vi "参数设置页.vi"() -> ()   [LabVIEW 2016, in "斯坦道氨氮.lvlib"]
uses:
  <vilib>/Plasmionique/MB Master/MB_Master/MB_Master.lvclass
  <vilib>/ptbypt/NI_PtbyPt.lvlib
panel:
  in  "简易流程路径":path=path "data/流程.xml"
  out "数据刷新时间":string
  in  "通讯连接":bool
  out "MB table":enum32{"Serial", "TCP"}(tab)
  in  "请选择串口:":refnum<visa-resource-name>
  in  "IP":string="127.0.0.1"
  in  "PORT":string="1001"
  in  "通信方式选择":enum16{"串口", "TCP"}(ring)
  in  "盐度自动补偿：":bool
  out "盐度补偿值":dbl caption="盐度补偿值："
  in  "刷新":bool
  in  "测量模式":T1(ring)
  in  "参数下拉列表":u16(ring) items=["总磷"=1, "总氮"=2]
  in  "量程下拉列表":enum16{"低量程", "高量程"}(ring)
  in  "测试流程路径":path=path "data/流程.xml"
  in  "标样核查量程模式":enum16{"高量程", "低量程", "自动"}(ring) caption="标样核查量程模式："
  in  "加标回收量程模式":enum16{"高量程", "低量程", "自动"}(ring) caption="加标回收量程模式："
  in  "跨度核查量程模式":enum16{"高量程", "低量程", "自动"}(ring) caption="跨度核查量程模式："
  in  "零点核查量程模式":enum16{"高量程", "低量程", "自动"}(ring) caption="零点核查量程模式："
  in  "水样测试量程模式":enum16{"高量程", "低量程", "自动"}(ring) caption="水样测试量程模式："
  out "稀释度":dbl caption="稀释度："
  out "阈值（高->低）":dbl caption="阈值（高->低）："
  out "阈值（低->高）":dbl caption="阈值（低->高）："
  out "量程下限":dbl caption="量程下限："
  out "量程上限":dbl caption="量程上限："
  out "检出限":dbl caption="检出限："
  out "曲线截距":dbl caption="曲线截距：" format="%#.6f"
  out "曲线斜率":dbl caption="曲线斜率：" format="%#.6f"
  out "二次多项式系数":dbl caption="二次多项式系数：" format="%#.6f"
  out "消解时长":dbl caption="消解时长："
  out "消解温度":dbl caption="消解温度："
  out "测量精度":u16 caption="测量精度："
  in  "标样核查标液浓度":dbl caption="标样核查标液浓度："
  in  "跨度核查标液浓度":dbl caption="跨度核查标液浓度："
  in  "零点核查标液浓度":dbl caption="零点核查标液浓度："
  in  "跨度值":dbl caption="跨度值："
  # "ppt"
  # "mg/L"
  # "mg/L"
  # "mg/L"
  # "mg/L"
  # "mg/L"
  # "min"
  # "℃"
  # "mg/L"
  # "mg/L"
  # "mg/L"
  # "mg/L"
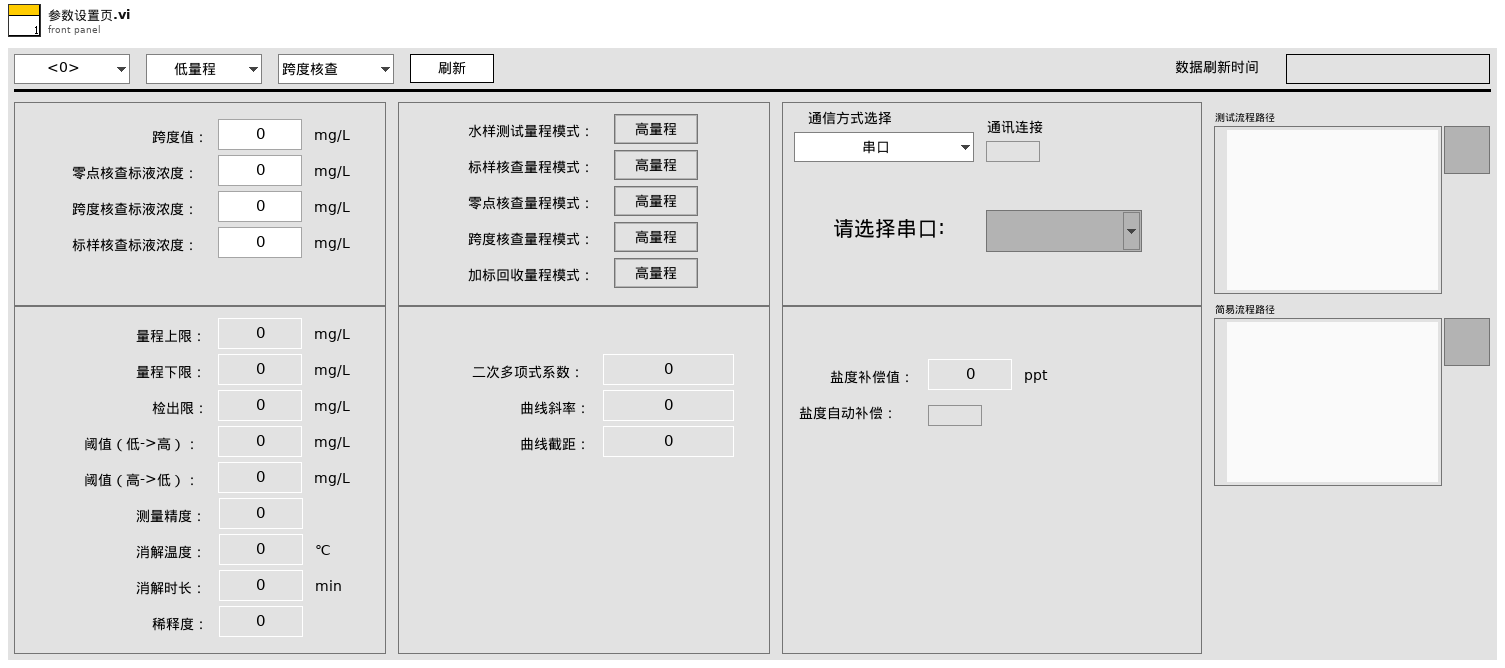
[diagram p1: front panel]
types:
  T1 = enum16{"跨度核查", "水样测量", "零点核查", "标样核查", "加标回收", "快捷测试", "空白校准", "标样校准"}
  T2 = typedef "LVStringsAndValuesArrayTypeDef_U16.ctl" = cluster{"String":string, "Value":u16}[]
  T3 = enum8{"Enabled", "Disabled", "Disabled and Grayed Out"}
  T4 = cluster{"标液浓度1":dbl, "测量吸光度1":dbl, "样品1启用":bool, "标液浓度2":dbl, "测量吸光度2":dbl, "样品2启用":bool, "标液浓度3":dbl, "测量吸光度3":dbl, "样品3启用":bool, "标液浓度4":dbl, "测量吸光度4":dbl, "样品4启用":bool, "标液浓度5":dbl, "测量吸光度5":dbl, "样品5启用":bool, "模型":enum32{"线性", "多项式"}, "精度":dbl, "XY图":cluster{"X Values":dbl[], "Y Values":dbl[]}[], "拟合公式":string, "r^2":dbl, "标样一校准时间":timestamp, "标样二校准时间":timestamp, "标样三校准时间":timestamp, "标样四校准时间":timestamp, "标样五校准时间":timestamp, "二次方程":cluster{"c":dbl, "x":dbl, "x^2":dbl}, "标定时间":timestamp}
  T5 = cluster{"系统时间":timestamp, "工作状态":u16, "测量模式":enum16{"待机", "连续模式", "周期模式", "定点模式", "受控模式", "手动模式"}, "告警代码":u16, "故障代码":u16, "日志代码":u16, "软件版本":u16, "F0":sgl, "F1":sgl, "F2":sgl, "F3":sgl, "T":sgl, "H":sgl, "id":u16, "flowid":u16, "量程":u16, "总磷控温温度1":sgl, "营养盐控温温度2":sgl, "ADC":sgl}
  T6 = cluster{"测量精度":u16, "检出限":dbl, "上限":dbl, "下限":dbl, "阈值（低->高）":dbl, "阈值（高->低）":dbl, "稀释度":dbl}
  T7 = cluster{"泵类型":u8, "进样速度":u32, "出样速度":u32, "泵阀量":u8, "光谱仪类型":u8, "光谱采样次数":u8, "氙灯次数":u8, "B":u16, "C":u16, "D":u16, "E":u16, "B_COD":u16, "C_COD":u16, "D_COD":u16, "E_COD":u16, "G":u16, "M":u16, "N":u16, "氨氮注射泵控温下限":sgl, "氨氮注射泵控温上限":sgl, "总氮注射泵控温下限":sgl, "总氮注射泵控温上限":sgl, "消解温度下限":sgl, "消解温度上限":sgl, "加热10s限值":sgl, "高温高压阀开阀温度":sgl, "总氮x公式0":u8, "总氮x公式1":sgl, "总氮x公式2":sgl, "总磷浊度稀释系数":sgl, "总磷浊度补偿权重1":sgl, "总磷浊度补偿权重2":sgl, "盐度系数":sgl, "氨氮补偿系数1":sgl, "氨氮补偿系数2":sgl}
  T8 = cluster{"标液浓度1":dbl, "测量吸光度1":dbl, "样品1启用":bool, "标液浓度2":dbl, "测量吸光度2":dbl, "样品2启用":bool, "标液浓度3":dbl, "测量吸光度3":dbl, "样品3启用":bool, "标液浓度4":dbl, "测量吸光度4":dbl, "样品4启用":bool, "标液浓度5":dbl, "测量吸光度5":dbl, "样品5启用":bool, "模型":enum32{"线性", "多项式"}, "精度":dbl, "XY图":cluster{"X Values":dbl[], "Y Values":dbl[]}[], "拟合公式":string, "r^2":dbl, "标样一校准时间":timestamp, "标样二校准时间":timestamp, "标样三校准时间":timestamp, "标样四校准时间":timestamp, "标样五校准时间":timestamp, "二次方程":cluster{"c":dbl, "x":dbl, "x^2":dbl}, "标定时间":timestamp}[][]
  T9 = typedef "斯坦道氨氮.lvlib/关键参数.ctl" = cluster{"测量量程":sgl, "测量检出限":sgl, "测量精度":sgl, "测量间隔":sgl, "消解温度":sgl, "消解时长":sgl, "三项式系数":sgl, "二次多项式系数":sgl, "曲线斜率":sgl, "曲线截距":sgl, "线性相关系数":sgl, "空白校准时间":timestamp, "标样校准时间":timestamp, "测量信号值":sgl, "稀释倍数":sgl, "量程系数":sgl}
  T10 = cluster{"水样测试量程模式":enum16{"高量程", "低量程", "自动"}, "零点核查量程模式":enum16{"高量程", "低量程", "自动"}, "跨度核查量程模式":enum16{"高量程", "低量程", "自动"}, "加标回收量程模式":enum16{"高量程", "低量程", "自动"}, "标样核查量程模式":enum16{"高量程", "低量程", "自动"}}
  T11 = cluster{"总磷跨度值":dbl, "总磷零点标准液浓度":dbl, "总磷跨度标准液浓度":dbl, "总磷标准液标准浓度":dbl, "总氮跨度值":dbl, "总氮零点标准液浓度":dbl, "总氮跨度标准液浓度":dbl, "总氮标准液标准浓度":dbl, "COD跨度值":dbl, "COD零点标准液浓度":dbl, "COD跨度标准液浓度":dbl, "COD标准液标准浓度":dbl, "氨氮跨度值":dbl, "氨氮零点标准液浓度":dbl, "氨氮跨度标准液浓度":dbl, "氨氮标准液标准浓度":dbl, "磷酸盐跨度值":dbl, "磷酸盐零点标准液浓度":dbl, "磷酸盐跨度标准液浓度":dbl, "磷酸盐标准液标准浓度":dbl, "硝氮跨度值":dbl, "硝氮零点标准液浓度":dbl, "硝氮跨度标准液浓度":dbl, "硝氮标准液标准浓度":dbl, "亚硝氮跨度值":dbl, "亚硝氮零点标准液浓度":dbl, "亚硝氮跨度标准液浓度":dbl, "亚硝氮标准液标准浓度":dbl, "硫化物跨度值":dbl, "硫化物零点标准液浓度":dbl, "硫化物跨度标准液浓度":dbl, "硫化物标准液标准浓度":dbl, "硅酸盐跨度值":dbl, "硅酸盐零点标准液浓度":dbl, "硅酸盐跨度标准液浓度":dbl, "硅酸盐标准液标准浓度":dbl}
  T12 = cluster{"水样测试量程模式":u16, "零点核查量程模式":u16, "跨度核查量程模式":u16, "加标回收量程模式":u16, "标样核查量程模式":u16}
  T13 = cluster{"水样测试量程模式":enum16{"H", "L", "AUTO"}, "空白核查量程模式":enum16{"H", "L", "AUTO"}, "跨度核查量程模式":enum16{"H", "L", "AUTO"}, "加标回收量程模式":enum16{"H", "L", "AUTO"}, "标样核查量程模式":enum16{"H", "L", "AUTO"}}
  T14 = cluster{"水样测试量程模式":u16, "空白核查量程模式":u16, "跨度核查量程模式":u16, "加标回收量程模式":u16, "标样核查量程模式":u16}
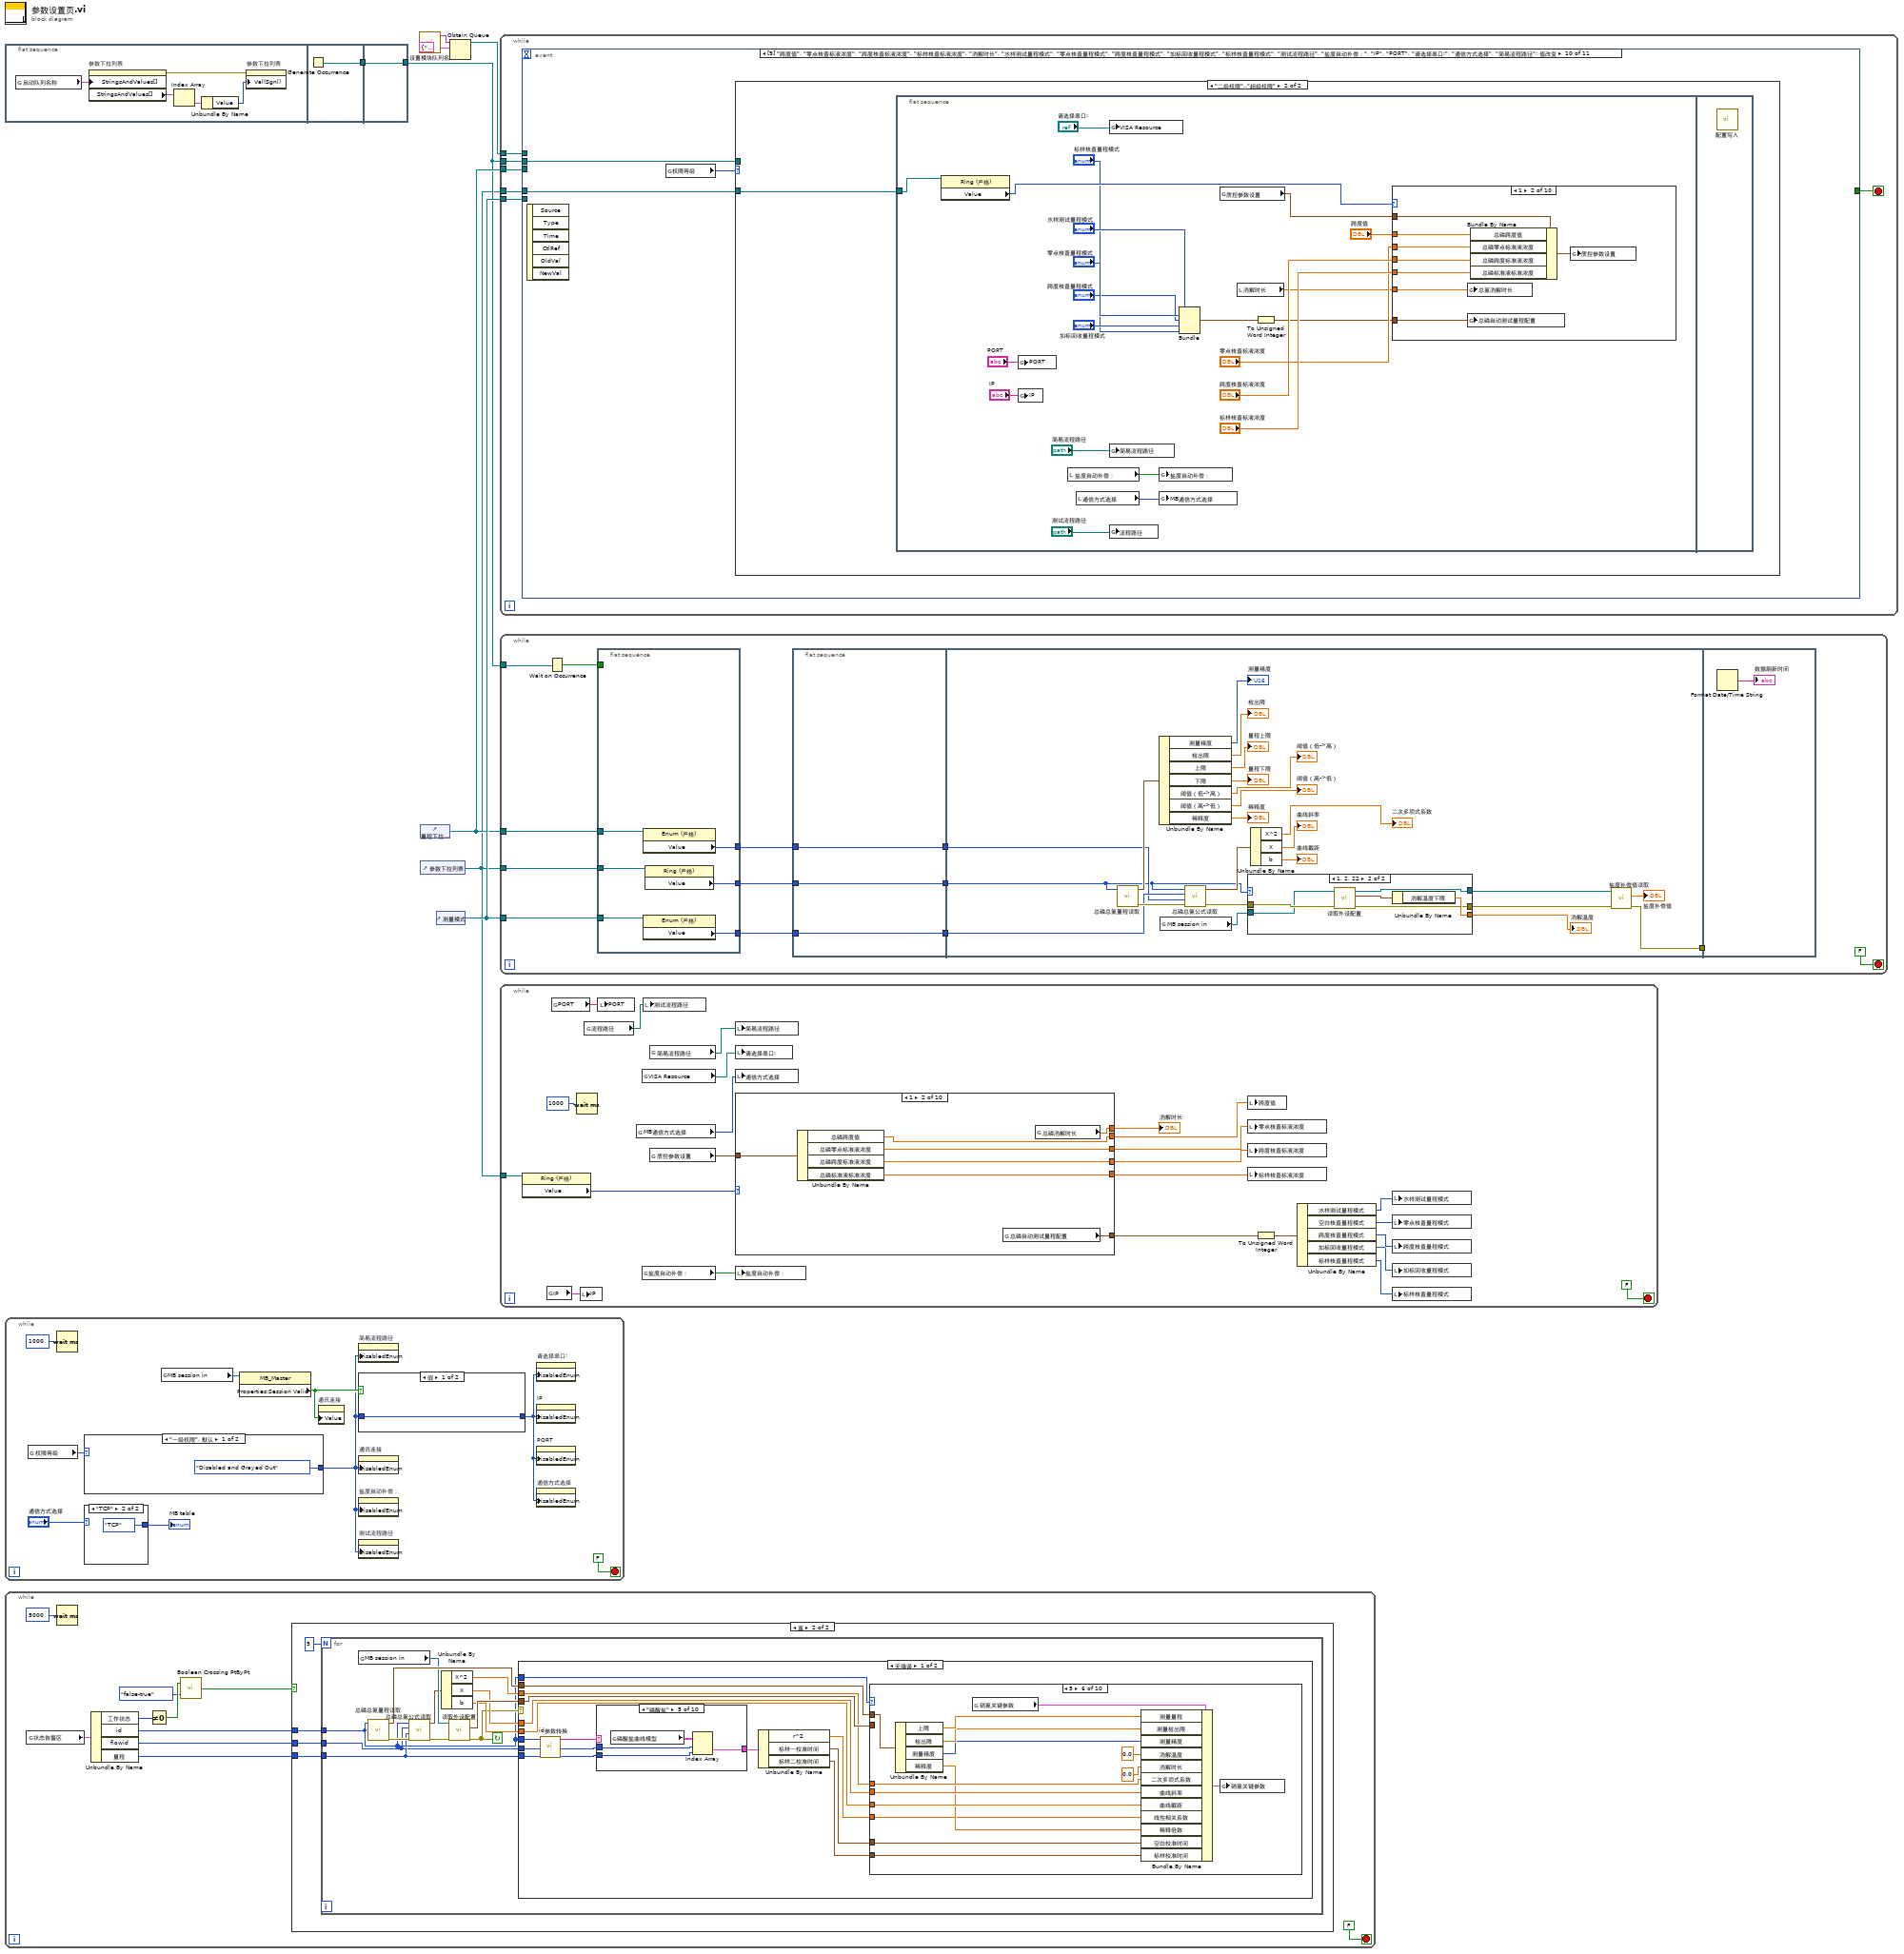
[diagram p0: block diagram]
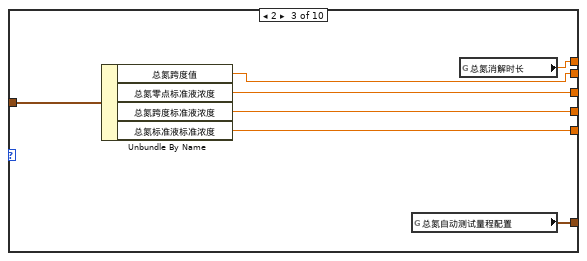
[diagram p3: hidden frame]
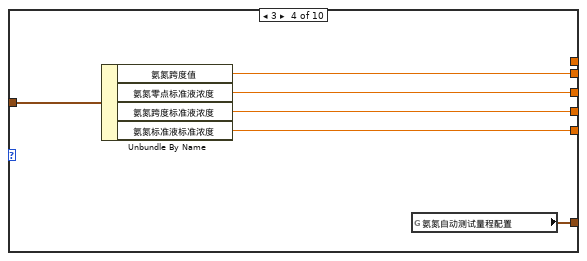
[diagram p4: hidden frame]
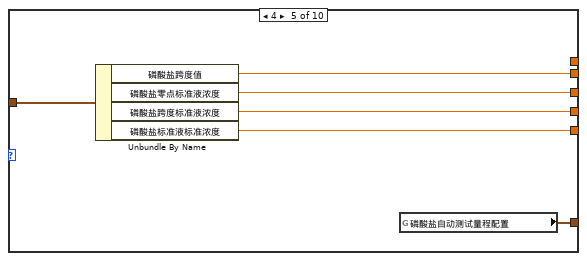
[diagram p5: hidden frame]
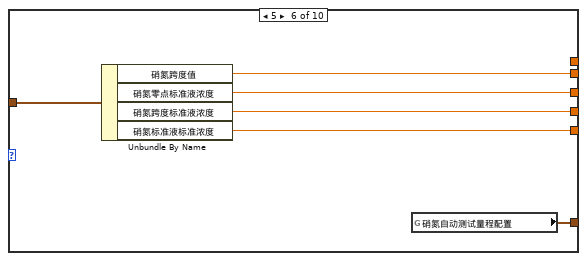
[diagram p6: hidden frame]
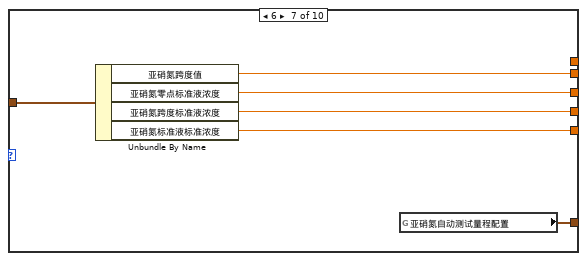
[diagram p7: hidden frame]
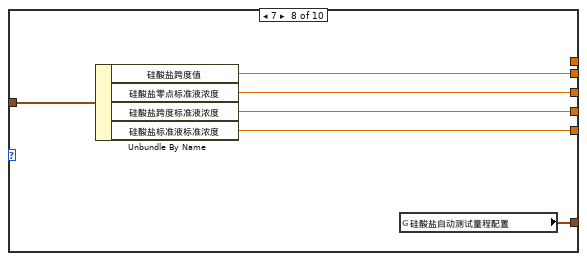
[diagram p8: hidden frame]
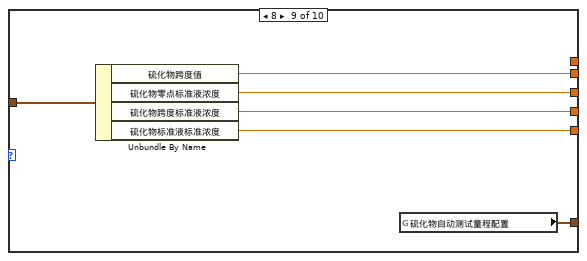
[diagram p9: hidden frame]
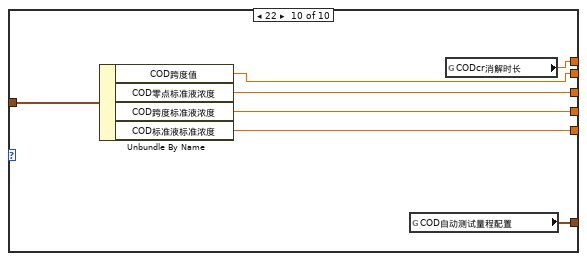
[diagram p10: hidden frame]
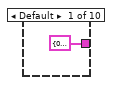
[diagram p12: hidden frame]
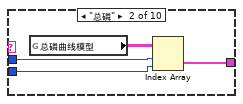
[diagram p13: hidden frame]
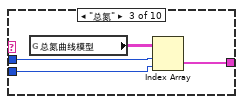
[diagram p14: hidden frame]
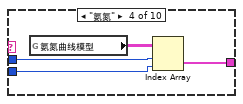
[diagram p15: hidden frame]
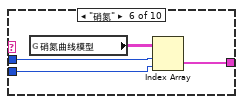
[diagram p16: hidden frame]
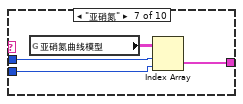
[diagram p17: hidden frame]
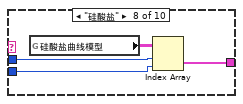
[diagram p18: hidden frame]
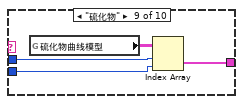
[diagram p19: hidden frame]
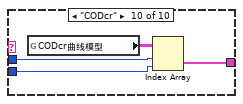
[diagram p20: hidden frame]
diagram:
  n1 = flat-sequence {
    tunnel: [w14] -> w8
    tunnel: [w15] -> w2
    tunnel: w8 -> [w15]
    frame #0 {
      n2 = global read "总磷总氮断电保存全局变量.vi" "启动队列名称"() -> (w9:cluster{"String":string, "Value":u16}[])
      n3 = property on="参数下拉列表" class="Ring (严格)"("StringsAndValues[]"=w9) -> (error out=w12:errorcluster, "StringsAndValues[]"=w10:T2)  [unwired: 2 in, 1 out]
      n4 = Index Array(array=w10) -> (element=w11:cluster{"String":string, "Value":u16})  [unwired: 1 in]
      n5 = Unbundle By Name(w11) -> ("Value"=w13:u16)
      n6 = property on="参数下拉列表" class="Ring (严格)"(error in=w12, "Val(Sgnl)"=w13) -> ()  [unwired: 1 in, 2 out]
    }
    frame #1 {
      n7 = Generate Occurrence() -> (w14:refnum<k4>)
    }
    frame #2 {
    }
  }
  n8 = while {
    stop <- FALSE stop-if-true
    n9 = global read "VAR总磷总氮全局变量.vi" "权限等级"() -> (w17:enum16{"一级权限", "二级权限", "三级权限", "超级权限"})
    n10 = Wait (ms)(milliseconds to wait=u32 1000 ("等待时间（毫秒）")) -> ()  [unwired: 1 out]
    n11 = case shown="\"一级权限\", 默认" w17 {
      tunnel: [T3."Disabled and Grayed Out" ("禁用") T3."Enabled" ("禁用")] -> w16
      frame "一级权限", Default {
      }
      frame "二级权限".."超级权限" {
      }
    }
    n12 = case shown="\"TCP\"" "通信方式选择" {
      tunnel: [enum32{"Serial", "TCP"}."Serial" ("MB table") enum32{"Serial", "TCP"}."TCP" ("MB table")] -> w19
      frame "串口", Default {
      }
      frame "TCP" {
      }
    }
    "MB table" <- w19
    n13 = global read "VAR总磷总氮全局变量.vi" "MB session in"() -> (w23:refnum<class "MB_Master.lvclass">)
    n14 = property class="MB_Master"(reference=w23) -> ("Properties:Session Valid"=w21:bool)  [unwired: 1 in, 2 out]
    n15 = property on="通讯连接" class="Bool (严格)"("Value"=w21) -> ()  [unwired: 2 in, 2 out]
    n16 = property on="简易流程路径" class="Path"("DisabledEnum"=w16) -> ()  [unwired: 2 in, 2 out]
    n17 = case shown="假" w21 {
      tunnel: [w29 T3."Disabled and Grayed Out" ("禁用")] -> w20
      tunnel: w16 -> [w29 _]
      frame False {
      }
      frame True {
      }
    }
    n18 = property on="通讯连接" class="Bool (严格)"("DisabledEnum"=w16) -> ()  [unwired: 2 in, 2 out]
    n19 = property on="盐度自动补偿：" class="Bool (严格)"("DisabledEnum"=w16) -> ()  [unwired: 2 in, 2 out]
    n20 = property on="测试流程路径" class="Path"("DisabledEnum"=w16) -> ()  [unwired: 2 in, 2 out]
    n21 = property on="请选择串口:" class="VISAName"("DisabledEnum"=w20) -> ()  [unwired: 2 in, 2 out]
    n22 = property on="IP" class="Str"("DisabledEnum"=w20) -> ()  [unwired: 2 in, 2 out]
    n23 = property on="PORT" class="Str"("DisabledEnum"=w20) -> ()  [unwired: 2 in, 2 out]
    n24 = property on="通信方式选择" class="Enum (严格)"("DisabledEnum"=w20) -> ()  [unwired: 2 in, 2 out]
  }
  n25 = while {
    stop <- FALSE stop-if-true
    n26 = global read "VAR总磷总氮全局变量.vi" "状态告警区"() -> (w40:T5)
    n27 = Wait (ms)(milliseconds to wait=u32 5000 ("等待时间（毫秒）")) -> ()  [unwired: 1 out]
    n28 = Unbundle By Name(w40) -> ("工作状态"=w36:u16, "id"=w37:u16, "flowid"=w38:u16, "量程"=w39:u16)
    n29 = Not Equal To 0?(x=w36) -> (x != 0?=w35:bool)
    n30 = call <vilib>:"Boolean Crossing PtByPt.vi"("direction"=enum16{"either", "false-true", "true-false"}."false-true", "input"=w35) -> ("crossing"=w33:bool)  [unwired: 1 in]
    n31 = case shown="真" w33 {
      tunnel: w39 -> [_ w44]
      tunnel: w38 -> [_ w43]
      tunnel: w37 -> [_ w42]
      frame False {
      }
      frame True {
        n32 = for {
          N: 5 -> [_]
          tunnel: w44 -> [w46]
          tunnel: w43 -> [w45]
          tunnel: w42 -> [w47]
          stop <- w48 continue-if-true
          n33 = global read "VAR总磷总氮全局变量.vi" "MB session in"() -> (w56:refnum<class "MB_Master.lvclass">)
          n34 = call "总磷总氮量程读取.vi"("测量参数"=w47) -> ("error out"=w50:errorcluster, "量程参数读取"=w57:T6)  [unwired: 9 in]
          n35 = call "总磷总氮公式读取.vi"("error in (no error)"=w50, "量程"=w46, "测量模式"=w45, "测量参数"=w47) -> ("error out"=w49:errorcluster, "公式"=w54:cluster{"X^2":dbl, "X":dbl, "b":dbl})  [unwired: 6 in]
          n36 = Unbundle By Name(w54) -> ("X^2"=w53:dbl, "X"=w52:dbl, "b"=w51:dbl)
          n37 = call "读取外设配置.vi"("error in (no error)"=w49, "MB session in"=w56) -> ("error out"=w48:errorcluster, "外设配置"=w55:T7)  [unwired: 7 in, 1 out]
          n38 = case shown="无错误" w48 {
            tunnel: w57 -> [w71 _]
            tunnel: w55 -> [w70 _]
            tunnel: w53 -> [w69 _]
            tunnel: w52 -> [w68 _]
            tunnel: w51 -> [w67 _]
            tunnel: w47 -> [w66 _]
            tunnel: w47 -> [w63 _]
            tunnel: w46 -> [w59 _]
            tunnel: w45 -> [w58 _]
            frame No Error {
              n39 = call "id参数转换.vi"("id"=w63) -> ("table输出"=w65:string)  [unwired: 9 in, 1 out]
              n40 = case shown="\"磷酸盐\"" w65 {
                tunnel: w59 -> [_ w75 w77 w82 w86 w90 w94 w98 w102 w106]
                tunnel: w58 -> [_ w76 w78 w83 w87 w91 w95 w99 w103 w107]
                tunnel: [T4 {"标液浓度1"=0.0, "测量吸光度1"=0.0, "样品1启用"=FALSE, "标液浓度2"=0.0, "测量吸光度2"=0.0, "样品2启用"=FALSE, "标液浓度3"=0.0, "测量吸光度3"=0.0, "样品3启用"=FALSE, "标液浓度4"=0.0, "测量吸光度4"=0.0, "样品4启用"=FALSE, "标液浓度5"=0.0, "测量吸光度5"=0.0, "样品5启用"=FALSE, "模型"=enum."线性", "精度"=0.0, "XY图"=[], "拟合公式"="", "r^2"=0.0, "标样一校准时间"=timestamp(0 s since 1904-01-01), "标样二校准时间"=timestamp(0 s since 1904-01-01), "标样三校准时间"=timestamp(0 s since 1904-01-01), "标样四校准时间"=timestamp(0 s since 1904-01-01), "标样五校准时间"=timestamp(0 s since 1904-01-01), "二次方程"={"c"=0.0, "x"=0.0, "x^2"=0.0}, "标定时间"=timestamp(0 s since 1904-01-01)} ("总磷曲线模型") w73 w79 w81 w85 w89 w93 w97 w101 w105] -> w64
                frame Default {
                }
                frame "总磷" {
                  n41 = global read "校准数据全局变量.vi" "总磷曲线模型"() -> (w74:T8)
                  n42 = Index Array(array=w74, index (row)=w76, index (col)=w75) -> (element=w73:T4)
                }
                frame "总氮" {
                  n43 = global read "校准数据全局变量.vi" "总氮曲线模型"() -> (w80:T8)
                  n44 = Index Array(array=w80, index (row)=w78, index (col)=w77) -> (element=w79:T4)
                }
                frame "氨氮" {
                  n45 = global read "校准数据全局变量.vi" "氨氮曲线模型"() -> (w84:T8)
                  n46 = Index Array(array=w84, index (row)=w83, index (col)=w82) -> (element=w81:T4)
                }
                frame "磷酸盐" {
                  n47 = global read "校准数据全局变量.vi" "磷酸盐曲线模型"() -> (w88:T8)
                  n48 = Index Array(array=w88, index (row)=w87, index (col)=w86) -> (element=w85:T4)
                }
                frame "硝氮" {
                  n49 = global read "校准数据全局变量.vi" "硝氮曲线模型"() -> (w92:T8)
                  n50 = Index Array(array=w92, index (row)=w91, index (col)=w90) -> (element=w89:T4)
                }
                frame "亚硝氮" {
                  n51 = global read "校准数据全局变量.vi" "亚硝氮曲线模型"() -> (w96:T8)
                  n52 = Index Array(array=w96, index (row)=w95, index (col)=w94) -> (element=w93:T4)
                }
                frame "硅酸盐" {
                  n53 = global read "校准数据全局变量.vi" "硅酸盐曲线模型"() -> (w100:T8)
                  n54 = Index Array(array=w100, index (row)=w99, index (col)=w98) -> (element=w97:T4)
                }
                frame "硫化物" {
                  n55 = global read "校准数据全局变量.vi" "硫化物曲线模型"() -> (w104:T8)
                  n56 = Index Array(array=w104, index (row)=w103, index (col)=w102) -> (element=w101:T4)
                }
                frame "CODcr" {
                  n57 = global read "校准数据全局变量.vi" "CODcr曲线模型"() -> (w108:T8)
                  n58 = Index Array(array=w108, index (row)=w107, index (col)=w106) -> (element=w105:T4)
                }
              }
              n59 = Unbundle By Name(w64) -> ("r^2"=w62:dbl, "标样一校准时间"=w61:timestamp, "标样二校准时间"=w60:timestamp)
              n60 = case shown="5" w66 {
                tunnel: w71 -> [_ w122 w138 w153 w168 w183 w196 w211 w226 w242]
                tunnel: w70 -> [_ w118 w134 _ _ _ _ _ _ w234]
                tunnel: w69 -> [_ w115 w131 w149 w164 w179 w192 w207 w222 w238]
                tunnel: w68 -> [_ w114 w130 w148 w163 w178 w191 w206 w221 w237]
                tunnel: w67 -> [_ w113 w129 w147 w162 w177 w190 w205 w220 w236]
                tunnel: w62 -> [_ w109 w127 w143 w156 w173 _ w201 w214 w231]
                tunnel: w61 -> [_ w110 w126 w142 w158 w172 _ w200 w216 w230]
                tunnel: w60 -> [_ w111 w125 w141 w157 w171 _ w199 w215 w229]
                frame 0, Default {
                }
                frame 1 {
                  n61 = Unbundle By Name(w118) -> ("消解温度下限"=w117:sgl)
                  n62 = Unbundle By Name(w122) -> ("上限"=w121:dbl, "检出限"=w120:dbl, "测量精度"=w119:u16, "稀释度"=w112:dbl)
                  n63 = global read "VAR总磷总氮全局变量.vi" "总磷关键参数"() -> (w123:T9)
                  n64 = global read "总磷总氮断电保存全局变量.vi" "总磷消解时长"() -> (w116:dbl)
                  n65 = Bundle By Name(cluster=w123, "测量量程"=w121, "测量检出限"=w120, "测量精度"=w119, "消解温度"=w117, "消解时长"=w116, "二次多项式系数"=w115, "曲线斜率"=w114, "曲线截距"=w113, "线性相关系数"=w109, "稀释倍数"=w112, "空白校准时间"=w110, "标样校准时间"=w111) -> (w124:T9)
                  n66 = global write "VAR总磷总氮全局变量.vi" "总磷关键参数"(w124) -> ()
                }
                frame 2 {
                  n67 = Unbundle By Name(w134) -> ("消解温度下限"=w133:sgl)
                  n68 = Unbundle By Name(w138) -> ("上限"=w137:dbl, "检出限"=w136:dbl, "测量精度"=w135:u16, "稀释度"=w128:dbl)
                  n69 = global read "VAR总磷总氮全局变量.vi" "总氮关键参数"() -> (w139:T9)
                  n70 = global read "总磷总氮断电保存全局变量.vi" "总氮消解时长"() -> (w132:dbl)
                  n71 = Bundle By Name(cluster=w139, "测量量程"=w137, "测量检出限"=w136, "测量精度"=w135, "消解温度"=w133, "消解时长"=w132, "二次多项式系数"=w131, "曲线斜率"=w130, "曲线截距"=w129, "线性相关系数"=w127, "稀释倍数"=w128, "空白校准时间"=w126, "标样校准时间"=w125) -> (w140:T9)
                  n72 = global write "VAR总磷总氮全局变量.vi" "总氮关键参数"(w140) -> ()
                }
                frame 3 {
                  n73 = Unbundle By Name(w153) -> ("上限"=w152:dbl, "检出限"=w151:dbl, "测量精度"=w150:u16, "稀释度"=w146:dbl)
                  n74 = global read "VAR总磷总氮全局变量.vi" "氨氮关键参数"() -> (w154:T9)
                  n75 = Bundle By Name(cluster=w154, "测量量程"=w152, "测量检出限"=w151, "测量精度"=w150, "消解温度"=sgl 0.0, "消解时长"=sgl 0.0, "二次多项式系数"=w149, "曲线斜率"=w148, "曲线截距"=w147, "线性相关系数"=w143, "稀释倍数"=w146, "空白校准时间"=w142, "标样校准时间"=w141) -> (w155:T9)
                  n76 = global write "VAR总磷总氮全局变量.vi" "氨氮关键参数"(w155) -> ()
                }
                frame 4 {
                  n77 = Unbundle By Name(w168) -> ("上限"=w167:dbl, "检出限"=w166:dbl, "测量精度"=w165:u16, "稀释度"=w161:dbl)
                  n78 = global read "VAR总磷总氮全局变量.vi" "磷酸盐关键参数"() -> (w169:T9)
                  n79 = Bundle By Name(cluster=w169, "测量量程"=w167, "测量检出限"=w166, "测量精度"=w165, "消解温度"=sgl 0.0, "消解时长"=sgl 0.0, "二次多项式系数"=w164, "曲线斜率"=w163, "曲线截距"=w162, "线性相关系数"=w156, "稀释倍数"=w161, "空白校准时间"=w158, "标样校准时间"=w157) -> (w170:T9)
                  n80 = global write "VAR总磷总氮全局变量.vi" "磷酸盐关键参数"(w170) -> ()
                }
                frame 5 {
                  n81 = Unbundle By Name(w183) -> ("上限"=w182:dbl, "检出限"=w181:dbl, "测量精度"=w180:u16, "稀释度"=w176:dbl)
                  n82 = global read "VAR总磷总氮全局变量.vi" "硝氮关键参数"() -> (w184:T9)
                  n83 = Bundle By Name(cluster=w184, "测量量程"=w182, "测量检出限"=w181, "测量精度"=w180, "消解温度"=sgl 0.0, "消解时长"=sgl 0.0, "二次多项式系数"=w179, "曲线斜率"=w178, "曲线截距"=w177, "线性相关系数"=w173, "稀释倍数"=w176, "空白校准时间"=w172, "标样校准时间"=w171) -> (w185:T9)
                  n84 = global write "VAR总磷总氮全局变量.vi" "硝氮关键参数"(w185) -> ()
                }
                frame 6 {
                  n85 = Unbundle By Name(w196) -> ("上限"=w195:dbl, "检出限"=w194:dbl, "测量精度"=w193:u16, "稀释度"=w188:dbl)
                  n86 = global read "VAR总磷总氮全局变量.vi" "亚硝氮关键参数"() -> (w197:T9)
                  n87 = Bundle By Name(cluster=w197, "测量量程"=w195, "测量检出限"=w194, "测量精度"=w193, "消解温度"=sgl 0.0, "消解时长"=sgl 0.0, "二次多项式系数"=w192, "曲线斜率"=w191, "曲线截距"=w190, "线性相关系数"=sgl 1.0, "稀释倍数"=w188) -> (w198:T9)
                  n88 = global write "VAR总磷总氮全局变量.vi" "亚硝氮关键参数"(w198) -> ()
                }
                frame 7 {
                  n89 = Unbundle By Name(w211) -> ("上限"=w210:dbl, "检出限"=w209:dbl, "测量精度"=w208:u16, "稀释度"=w204:dbl)
                  n90 = global read "VAR总磷总氮全局变量.vi" "硅酸盐关键参数"() -> (w212:T9)
                  n91 = Bundle By Name(cluster=w212, "测量量程"=w210, "测量检出限"=w209, "测量精度"=w208, "消解温度"=sgl 0.0, "消解时长"=sgl 0.0, "二次多项式系数"=w207, "曲线斜率"=w206, "曲线截距"=w205, "线性相关系数"=w201, "稀释倍数"=w204, "空白校准时间"=w200, "标样校准时间"=w199) -> (w213:T9)
                  n92 = global write "VAR总磷总氮全局变量.vi" "硅酸盐关键参数"(w213) -> ()
                }
                frame 8 {
                  n93 = Unbundle By Name(w226) -> ("上限"=w225:dbl, "检出限"=w224:dbl, "测量精度"=w223:u16, "稀释度"=w219:dbl)
                  n94 = global read "VAR总磷总氮全局变量.vi" "硫化物关键参数"() -> (w227:T9)
                  n95 = Bundle By Name(cluster=w227, "测量量程"=w225, "测量检出限"=w224, "测量精度"=w223, "消解温度"=sgl 0.0, "消解时长"=sgl 0.0, "二次多项式系数"=w222, "曲线斜率"=w221, "曲线截距"=w220, "线性相关系数"=w214, "稀释倍数"=w219, "空白校准时间"=w216, "标样校准时间"=w215) -> (w228:T9)
                  n96 = global write "VAR总磷总氮全局变量.vi" "硫化物关键参数"(w228) -> ()
                }
                frame 22 {
                  n97 = Unbundle By Name(w234) -> ("消解温度下限"=w233:sgl)
                  n98 = Unbundle By Name(w242) -> ("上限"=w241:dbl, "检出限"=w240:dbl, "测量精度"=w239:u16, "稀释度"=w235:dbl)
                  n99 = global read "VAR总磷总氮全局变量.vi" "CODcr关键参数"() -> (w243:T9)
                  n100 = global read "总磷总氮断电保存全局变量.vi" "CODcr消解时长"() -> (w232:dbl)
                  n101 = Bundle By Name(cluster=w243, "测量量程"=w241, "测量检出限"=w240, "测量精度"=w239, "消解温度"=w233, "消解时长"=w232, "二次多项式系数"=w238, "曲线斜率"=w237, "曲线截距"=w236, "线性相关系数"=w231, "稀释倍数"=w235, "空白校准时间"=w230, "标样校准时间"=w229) -> (w244:T9)
                  n102 = global write "VAR总磷总氮全局变量.vi" "CODcr关键参数"(w244) -> ()
                }
              }
            }
            frame Error {
            }
          }
        }
      }
    }
  }
  n103 = call "设置模块队列名.vi"() -> ("Msg"=w6:string)  [unwired: 5 in]
  n104 = control-ref of="量程下拉列表"() -> (w3:refnum<vi>)
  n105 = control-ref of="参数下拉列表"() -> (w1:refnum<vi>)
  n106 = control-ref of="测量模式"() -> (w4:refnum<vi>)
  n107 = Obtain Queue(name (unnamed)=w6, element data type=cluster{"命令":string, "data":variant} {"命令"="", "data"=variant}) -> (queue out=w5:refnum<queue>)  [unwired: 3 in, 2 out]
  n108 = while {
    tunnel: w2 -> [w249]
    tunnel: w1 -> [w248]
    tunnel: w5 -> [w247]
    tunnel: w4 -> [w246]
    tunnel: w3 -> [w245]
    stop <- w250 stop-if-true
    n109 = event shown="[9] \"跨度值\", \"零点核查标液浓度\", \"跨度核查标液浓度\", \"标样核查标液浓度\", \"消解时长\", \"水样测试量程模式\", \"零点核查量程模式\", \"跨度核查量程模式\", \"加标回收量程模式\", \"标样核查量程模式\", \"测试流程路径\", \"盐度自动补偿：\", \"IP\", \"PORT\", \"请选择串口:\", \"通信方式选择\", \"简易流程路径\": 值改变" {
      selector: _ -> [_ _ _ _ _ _ _ _ _ _ _]
      dyn-events: _ -> [_ _ _ _ _ _ _ _ _ _ _]
      timeout: _ -> [_ _ _ _ _ _ _ _ _ _ _]
      tunnel: [_ TRUE _ _ _ _ _ _ _ _ _] -> w250
      tunnel: w249 -> [_ _ w252 _ _ _ _ _ _ w299 _]
      tunnel: w248 -> [_ _ _ _ w271 _ _ _ _ w301 _]
      tunnel: w247 -> [_ _ _ _ _ _ _ _ _ _ w392]
      tunnel: w246 -> [_ _ _ _ _ _ _ _ _ _ _]
      tunnel: w245 -> [_ _ _ _ _ _ _ _ _ _ _]
      event Timeout {
        n110 = event-data() -> ()  [unwired: 1 in, 3 out]
      }
      event Panel Close {
        n111 = event-data() -> ()  [unwired: 1 in, 4 out]
      }
      event "参数下拉列表", "量程下拉列表", "测量模式", "刷新": Value Change {
        n112 = event-data() -> ()  [unwired: 1 in, 6 out]
        n113 = Set Occurrence(w252) -> ()
      }
      event "跨度值", "零点核查标液浓度", "跨度核查标液浓度", "标样核查标液浓度", "消解温度", "消解时长", "检出限", "量程上限", "量程下限", "阈值（低->高）", "阈值（高->低）", "稀释度": Mouse Down {
        n114 = event-data() -> ("CtlRef"=w254:refnum<vi>)  [unwired: 1 in, 5 out]
        n115 = global read "VAR总磷总氮全局变量.vi" "权限等级"() -> (w253:enum16{"一级权限", "二级权限", "三级权限", "超级权限"})
        n116 = case shown="\"二级权限\"..\"超级权限\"" w253 {
          tunnel: w254 -> [_ w258]
          frame "一级权限", Default {
          }
          frame "二级权限".."超级权限" {
            n117 = property class="DigNum (严格)"(reference=w258) -> (reference out=w256:refnum<vi>, "Value"=w257:dbl)  [unwired: 1 in, 1 out]
            n118 = call "数字键盘.vi"("OldNumber"=w257) -> ("NewNumber"=w255:dbl)
            n119 = property class="DigNum (严格)"(reference=w256, "Val(Sgnl)"=w255) -> ()  [unwired: 1 in, 2 out]
          }
        }
      }
      event "测量精度", "检出限", "量程上限", "量程下限", "阈值（低->高）", "阈值（高->低）", "稀释度": Value Change {
        n120 = event-data() -> ()  [unwired: 1 in, 6 out]
        n121 = property class="Ring (严格)"(reference=w271) -> ("Value"=w270:u16)  [unwired: 1 in, 2 out]
        n122 = local read "阈值（低->高）"() -> (w264:dbl)
        n123 = local read "阈值（高->低）"() -> (w263:dbl)
        n124 = local read "测量精度"() -> (w261:u16)
        n125 = local read "量程下限"() -> (w266:dbl)
        n126 = local read "量程上限"() -> (w267:dbl)
        n127 = local read "稀释度"() -> (w262:dbl)
        n128 = local read "检出限"() -> (w265:dbl)
        n129 = Bundle By Name(cluster=T6 {"测量精度"=0, "检出限"=0.0, "上限"=0.0, "下限"=0.0, "阈值（低->高）"=0.0, "阈值（高->低）"=0.0, "稀释度"=0.0} ("量程参数写入"), "测量精度"=w261, "检出限"=w265, "上限"=w267, "下限"=w266, "阈值（低->高）"=w264, "阈值（高->低）"=w263, "稀释度"=w262) -> (w268:T6)
        n130 = call "总磷总氮量程写入.vi"("量程参数写入"=w268, "测量参数"=w270) -> ("error out"=w259:errorcluster)  [unwired: 8 in]
        n131 = case shown="错误" w259 {
          tunnel: ["写入成功" "写入失败"] -> w260
          frame No Error {
          }
          frame Error {
          }
        }
        n132 = One Button Dialog(message=w260) -> ()  [unwired: 1 in, 1 out]
      }
      event "消解温度": Value Change {
        n133 = event-data() -> ("NewVal"=w276:dbl)  [unwired: 1 in, 5 out]
        n134 = global read "VAR总磷总氮全局变量.vi" "MB session in"() -> (w277:refnum<class "MB_Master.lvclass">)
        n135 = call "读取外设配置.vi"("MB session in"=w277) -> ("error out"=w280:errorcluster, "外设配置"=w279:T7)  [unwired: 8 in, 1 out]
        n136 = Bundle By Name(cluster=w279, "消解温度下限"=w276) -> (w278:T7)
        n137 = call "写入外设配置.vi"("error in (no error)"=w280, "外设配置"=w278, "MB session in"=w277) -> ("error out"=w275:errorcluster)  [unwired: 7 in, 1 out]
        n138 = case shown="错误" w275 {
          tunnel: ["写入成功" "写入失败"] -> w274
          frame No Error {
          }
          frame Error {
          }
        }
        n139 = One Button Dialog(message=w274) -> ()  [unwired: 1 in, 1 out]
      }
      event "测量精度": Mouse Down {
        n140 = event-data() -> ("CtlRef"=w284:refnum<vi>)  [unwired: 1 in, 7 out]
        n141 = global read "VAR总磷总氮全局变量.vi" "权限等级"() -> (w283:enum16{"一级权限", "二级权限", "三级权限", "超级权限"})
        n142 = case shown="\"二级权限\"..\"超级权限\"" w283 {
          tunnel: w284 -> [_ w288]
          frame "一级权限", Default {
          }
          frame "二级权限".."超级权限" {
            n143 = property class="DigNum (严格)"(reference=w288) -> (reference out=w286:refnum<vi>, "Value"=w287:u16)  [unwired: 1 in, 1 out]
            n144 = call "数字键盘.vi"("OldNumber"=w287) -> ("NewNumber"=w285:dbl)
            n145 = property class="DigNum (严格)"(reference=w286, "Val(Sgnl)"=w285) -> ()  [unwired: 1 in, 2 out]
          }
        }
      }
      event "盐度补偿值": Mouse Down {
        n146 = event-data() -> ("CtlRef"=w290:refnum<vi>)  [unwired: 1 in, 3 out]
        n147 = global read "VAR总磷总氮全局变量.vi" "权限等级"() -> (w289:enum16{"一级权限", "二级权限", "三级权限", "超级权限"})
        n148 = case shown="\"二级权限\"..\"超级权限\"" w289 {
          tunnel: w290 -> [_ w292]
          frame "一级权限", Default {
          }
          frame "二级权限".."超级权限" {
            n149 = case shown="假" "盐度自动补偿：" {
              tunnel: w292 -> [w296 _]
              frame False {
                n150 = property class="DigNum (严格)"(reference=w296) -> (reference out=w294:refnum<vi>, "Value"=w295:dbl)  [unwired: 1 in, 1 out]
                n151 = call "数字键盘.vi"("OldNumber"=w295) -> ("NewNumber"=w293:dbl)
                n152 = property class="DigNum (严格)"(reference=w294, "Val(Sgnl)"=w293) -> ()  [unwired: 1 in, 2 out]
              }
              frame True {
              }
            }
          }
        }
      }
      event "盐度补偿值": Value Change {
        n153 = event-data() -> ("NewVal"=w297:dbl)  [unwired: 1 in, 5 out]
        n154 = global read "VAR总磷总氮全局变量.vi" "MB session in"() -> (w298:refnum<class "MB_Master.lvclass">)
        n155 = call "盐度补偿值写入.vi"("盐度补偿值"=w297, "MB session in"=w298) -> ()  [unwired: 8 in, 2 out]
      }
      event "跨度值", "零点核查标液浓度", "跨度核查标液浓度", "标样核查标液浓度", "消解时长", "水样测试量程模式", "零点核查量程模式", "跨度核查量程模式", "加标回收量程模式", "标样核查量程模式", "测试流程路径", "盐度自动补偿：", "IP", "PORT", "请选择串口:", "通信方式选择", "简易流程路径": Value Change {
        n156 = event-data() -> ()  [unwired: 1 in, 6 out]
        n157 = global read "VAR总磷总氮全局变量.vi" "权限等级"() -> (w300:enum16{"一级权限", "二级权限", "三级权限", "超级权限"})
        n158 = case shown="\"二级权限\"..\"超级权限\"" w300 {
          tunnel: w301 -> [_ w303]
          tunnel: w299 -> [w302 _]
          frame "一级权限", Default {
            n159 = Set Occurrence(w302) -> ()
          }
          frame "二级权限".."超级权限" {
            n160 = flat-sequence {
              tunnel: w303 -> [w324]
              frame #0 {
                n161 = property class="Ring (严格)"(reference=w324) -> ("Value"=w323:u16)  [unwired: 1 in, 2 out]
                n162 = global write "总磷总氮断电保存全局变量.vi" "PORT"("PORT") -> ()
                n163 = global write "总磷总氮断电保存全局变量.vi" "IP"("IP") -> ()
                n164 = local read "盐度自动补偿："() -> (w310:bool)
                n165 = local read "通信方式选择"() -> (w306:enum16{"串口", "TCP"})
                n166 = global write "总磷总氮断电保存全局变量.vi" "VISA Resource"("请选择串口:") -> ()
                n167 = global write "总磷总氮断电保存全局变量.vi" "简易流程路径"("简易流程路径") -> ()
                n168 = global write "总磷总氮断电保存全局变量.vi" "流程路径"("测试流程路径") -> ()
                n169 = global write "总磷总氮断电保存全局变量.vi" "盐度自动补偿："(w310) -> ()
                n170 = global write "总磷总氮断电保存全局变量.vi" "MB通信方式选择"(w306) -> ()
                n171 = Bundle("水样测试量程模式"="水样测试量程模式", "零点核查量程模式"="零点核查量程模式", "跨度核查量程模式"="跨度核查量程模式", "加标回收量程模式"="加标回收量程模式", "标样核查量程模式"="标样核查量程模式") -> (w312:T10)  [unwired: 1 in]
                n172 = global read "总磷总氮断电保存全局变量.vi" "质控参数设置"() -> (w318:T11)
                n173 = local read "消解时长"() -> (w305:dbl)
                n174 = To Unsigned Word Integer(number=w312) -> (unsigned 16bit integer=w311:T12)
                n175 = case shown="1" w323 {
                  tunnel: "跨度值" -> [_ w331 w339 w346 w353 w360 w367 w374 w381 w388]
                  tunnel: "标样核查标液浓度" -> [_ w328 w336 w343 w350 w357 w364 w371 w378 w385]
                  tunnel: "跨度核查标液浓度" -> [_ w329 w337 w344 w351 w358 w365 w372 w379 w386]
                  tunnel: "零点核查标液浓度" -> [_ w330 w338 w345 w352 w359 w366 w373 w380 w387]
                  tunnel: w318 -> [_ w333 w341 w348 w355 w362 w369 w376 w383 w390]
                  tunnel: w311 -> [_ w327 w335 w342 w349 w356 w363 w370 w377 _]
                  tunnel: w305 -> [_ w326 w334 _ _ _ _ _ _ w384]
                  frame 0, Default {
                  }
                  frame 1 {
                    n176 = global write "总磷总氮断电保存全局变量.vi" "总氮消解时长"(w326) -> ()
                    n177 = global write "总磷总氮断电保存全局变量.vi" "总磷自动测试量程配置"(w327) -> ()
                    n178 = Bundle By Name(cluster=w333, "总磷跨度值"=w331, "总磷零点标准液浓度"=w330, "总磷跨度标准液浓度"=w329, "总磷标准液标准浓度"=w328) -> (w332:T11)
                    n179 = global write "总磷总氮断电保存全局变量.vi" "质控参数设置"(w332) -> ()
                  }
                  frame 2 {
                    n180 = global write "总磷总氮断电保存全局变量.vi" "总氮消解时长"(w334) -> ()
                    n181 = global write "总磷总氮断电保存全局变量.vi" "总氮自动测试量程配置"(w335) -> ()
                    n182 = Bundle By Name(cluster=w341, "总氮跨度值"=w339, "总氮零点标准液浓度"=w338, "总氮跨度标准液浓度"=w337, "总氮标准液标准浓度"=w336) -> (w340:T11)
                    n183 = global write "总磷总氮断电保存全局变量.vi" "质控参数设置"(w340) -> ()
                  }
                  frame 3 {
                    n184 = global write "总磷总氮断电保存全局变量.vi" "氨氮自动测试量程配置"(w342) -> ()
                    n185 = Bundle By Name(cluster=w348, "氨氮跨度值"=w346, "氨氮零点标准液浓度"=w345, "氨氮跨度标准液浓度"=w344, "氨氮标准液标准浓度"=w343) -> (w347:T11)
                    n186 = global write "总磷总氮断电保存全局变量.vi" "质控参数设置"(w347) -> ()
                  }
                  frame 4 {
                    n187 = Bundle By Name(cluster=w355, "磷酸盐跨度值"=w353, "磷酸盐零点标准液浓度"=w352, "磷酸盐跨度标准液浓度"=w351, "磷酸盐标准液标准浓度"=w350) -> (w354:T11)
                    n188 = global write "总磷总氮断电保存全局变量.vi" "磷酸盐自动测试量程配置"(w349) -> ()
                    n189 = global write "总磷总氮断电保存全局变量.vi" "质控参数设置"(w354) -> ()
                  }
                  frame 5 {
                    n190 = global write "总磷总氮断电保存全局变量.vi" "硝氮自动测试量程配置"(w356) -> ()
                    n191 = Bundle By Name(cluster=w362, "硝氮跨度值"=w360, "硝氮零点标准液浓度"=w359, "硝氮跨度标准液浓度"=w358, "硝氮标准液标准浓度"=w357) -> (w361:T11)
                    n192 = global write "总磷总氮断电保存全局变量.vi" "质控参数设置"(w361) -> ()
                  }
                  frame 6 {
                    n193 = Bundle By Name(cluster=w369, "亚硝氮跨度值"=w367, "亚硝氮零点标准液浓度"=w366, "亚硝氮跨度标准液浓度"=w365, "亚硝氮标准液标准浓度"=w364) -> (w368:T11)
                    n194 = global write "总磷总氮断电保存全局变量.vi" "亚硝氮自动测试量程配置"(w363) -> ()
                    n195 = global write "总磷总氮断电保存全局变量.vi" "质控参数设置"(w368) -> ()
                  }
                  frame 7 {
                    n196 = Bundle By Name(cluster=w376, "硅酸盐跨度值"=w374, "硅酸盐零点标准液浓度"=w373, "硅酸盐跨度标准液浓度"=w372, "硅酸盐标准液标准浓度"=w371) -> (w375:T11)
                    n197 = global write "总磷总氮断电保存全局变量.vi" "硅酸盐自动测试量程配置"(w370) -> ()
                    n198 = global write "总磷总氮断电保存全局变量.vi" "质控参数设置"(w375) -> ()
                  }
                  frame 8 {
                    n199 = Bundle By Name(cluster=w383, "硫化物跨度值"=w381, "硫化物零点标准液浓度"=w380, "硫化物跨度标准液浓度"=w379, "硫化物标准液标准浓度"=w378) -> (w382:T11)
                    n200 = global write "总磷总氮断电保存全局变量.vi" "硫化物自动测试量程配置"(w377) -> ()
                    n201 = global write "总磷总氮断电保存全局变量.vi" "质控参数设置"(w382) -> ()
                  }
                  frame 22 {
                    n202 = global write "总磷总氮断电保存全局变量.vi" "CODcr消解时长"(w384) -> ()
                    n203 = Bundle By Name(cluster=w390, "COD跨度值"=w388, "COD零点标准液浓度"=w387, "COD跨度标准液浓度"=w386, "COD标准液标准浓度"=w385) -> (w389:T11)
                    n204 = global write "总磷总氮断电保存全局变量.vi" "质控参数设置"(w389) -> ()
                  }
                }
              }
              frame #1 {
                n205 = call "配置写入.vi"() -> ()  [unwired: 11 in, 1 out]
              }
            }
          }
        }
      }
      event "通讯连接": Value Change {
        n206 = event-data() -> ("NewVal"=w391:bool)  [unwired: 1 in, 5 out]
        n207 = Flush Queue(queue=w392) -> (queue out=w393:refnum<queue>)  [unwired: 1 in, 2 out]
        n208 = case shown="假" w391 {
          tunnel: w393 -> [w394 w396]
          frame False {
            n209 = Enqueue Element(queue=w394, element=cluster{"命令":string, "data":variant} {"命令"="停用模块", "data"=variant} ("元素")) -> ()  [unwired: 2 in, 3 out]
          }
          frame True {
            n210 = Enqueue Element(queue=w396, element=cluster{"命令":string, "data":variant} {"命令"="启用模块", "data"=variant} ("元素")) -> ()  [unwired: 2 in, 3 out]
          }
        }
      }
    }
  }
  n211 = while {
    tunnel: w1 -> [w409]
    tunnel: w3 -> [w408]
    tunnel: w4 -> [w407]
    tunnel: w2 -> [w406]
    stop <- FALSE stop-if-true
    n212 = Wait on Occurrence(2:w406) -> (0:w400:bool)  [unwired: 2 in]
    n213 = flat-sequence {
      tunnel: w409 -> [w416]
      tunnel: w408 -> [w415]
      tunnel: w407 -> [w414]
      tunnel: [w413] -> w403
      tunnel: [w412] -> w402
      tunnel: [w411] -> w401
      tunnel: w400 -> [_]
      frame #0 {
        n214 = property class="Enum (严格)"(reference=w415) -> ("Value"=w412:enum16{"低量程", "高量程"})  [unwired: 1 in, 2 out]
        n215 = property class="Enum (严格)"(reference=w414) -> ("Value"=w411:T1)  [unwired: 1 in, 2 out]
        n216 = property class="Ring (严格)"(reference=w416) -> ("Value"=w413:u16)  [unwired: 1 in, 2 out]
      }
    }
    n217 = flat-sequence {
      tunnel: [w419] -> w405
      tunnel: [w418] -> w404
      tunnel: w403 -> [w417]
      tunnel: w402 -> [w419]
      tunnel: w401 -> [w418]
      tunnel: [w417] -> w398
      tunnel: w405 -> [w428]
      tunnel: w404 -> [w429]
      tunnel: [w422] -> w399
      tunnel: w398 -> [w421]
      tunnel: w399 -> [_]
      frame #0 {
      }
      frame #1 {
        n218 = call "总磷总氮量程读取.vi"("测量参数"=w421) -> ("error out"=w434:errorcluster, "量程参数读取"=w442:T6)  [unwired: 9 in]
        n219 = Unbundle By Name(w442) -> ("测量精度"=→"测量精度":u16, "检出限"=→"检出限":dbl, "上限"=→"量程上限":dbl, "下限"=→"量程下限":dbl, "阈值（低->高）"=→"阈值（低->高）":dbl, "阈值（高->低）"=→"阈值（高->低）":dbl, "稀释度"=→"稀释度":dbl)
        n220 = global read "VAR总磷总氮全局变量.vi" "MB session in"() -> (w420:refnum<class "MB_Master.lvclass">)
        n221 = call "总磷总氮公式读取.vi"("error in (no error)"=w434, "量程"=w428, "测量模式"=w429, "测量参数"=w421) -> ("error out"=w423:errorcluster, "公式"=w433:cluster{"X^2":dbl, "X":dbl, "b":dbl})  [unwired: 6 in]
        n222 = case shown="1, 2, 22" w421 {
          tunnel: [w444 w450] -> w427
          tunnel: [_ w448] -> w426
          tunnel: [w443 w447] -> w425
          tunnel: w423 -> [w443 w446]
          tunnel: w420 -> [w444 w445]
          frame 0, Default {
          }
          frame 1, 2, 22 {
            n223 = call "读取外设配置.vi"("error in (no error)"=w446, "MB session in"=w445) -> ("error out"=w447:errorcluster, "外设配置"=w449:T7, "MB session out"=w450:refnum<class "MB_Master.lvclass">)  [unwired: 7 in]
            n224 = Unbundle By Name(w449) -> ("消解温度下限"=w448:sgl)
          }
        }
        "消解温度" <- w426
        n225 = Unbundle By Name(w433) -> ("X^2"=→"二次多项式系数":dbl, "X"=→"曲线斜率":dbl, "b"=→"曲线截距":dbl)
        n226 = call "盐度补偿值读取.vi"("Error in"=w425, "MB session in"=w427) -> ("error out"=w422:errorcluster, "盐度补偿值"=→"盐度补偿值":sgl)  [unwired: 7 in, 1 out]
      }
      frame #2 {
        n227 = Format Date/Time String() -> (date/time string=→"数据刷新时间":string)  [unwired: 3 in]
      }
    }
  }
  n228 = while {
    tunnel: w1 -> [w454]
    stop <- FALSE stop-if-true
    n229 = property class="Ring (严格)"(reference=w454) -> ("Value"=w453:u16)  [unwired: 1 in, 2 out]
    n230 = global read "总磷总氮断电保存全局变量.vi" "IP"() -> (w471:string)
    n231 = global read "总磷总氮断电保存全局变量.vi" "PORT"() -> (w472:string)
    n232 = Wait (ms)(milliseconds to wait=u32 1000 ("等待时间（毫秒）")) -> ()  [unwired: 1 out]
    n233 = local write "IP"(w471) -> ()
    n234 = global read "总磷总氮断电保存全局变量.vi" "流程路径"() -> (w470:path)
    n235 = local write "PORT"(w472) -> ()
    n236 = global read "总磷总氮断电保存全局变量.vi" "MB通信方式选择"() -> (w468:enum16{"串口", "TCP"})
    n237 = global read "总磷总氮断电保存全局变量.vi" "VISA Resource"() -> (w473:refnum<visa-resource-name>)
    n238 = global read "总磷总氮断电保存全局变量.vi" "盐度自动补偿："() -> (w469:bool)
    n239 = local write "测试流程路径"(w470) -> ()
    n240 = global read "总磷总氮断电保存全局变量.vi" "简易流程路径"() -> (w452:path)
    n241 = global read "总磷总氮断电保存全局变量.vi" "质控参数设置"() -> (w463:T11)
    n242 = local write "简易流程路径"(w452) -> ()
    n243 = local write "请选择串口:"(w473) -> ()
    n244 = local write "通信方式选择"(w468) -> ()
    n245 = case shown="1" w453 {
      tunnel: [_ w482 w489 w495 w501 w507 w513 w519 w525 w532] -> w461
      tunnel: [_ w481 w488 _ _ _ _ _ _ w531] -> w462
      tunnel: w463 -> [_ w480 w487 w494 w500 w506 w512 w518 w524 w530]
      tunnel: [_ w479 w486 w493 w499 w505 w511 w517 w523 w529] -> w464
      tunnel: [_ w478 w485 w492 w498 w504 w510 w516 w522 w528] -> w465
      tunnel: [_ w477 w484 w491 w497 w503 w509 w515 w521 w527] -> w466
      tunnel: [_ w476 w483 w490 w496 w502 w508 w514 w520 w526] -> w467
      frame Default {
      }
      frame 1 {
        n246 = Unbundle By Name(w480) -> ("总磷跨度值"=w479:dbl, "总磷零点标准液浓度"=w478:dbl, "总磷跨度标准液浓度"=w477:dbl, "总磷标准液标准浓度"=w476:dbl)
        n247 = global read "总磷总氮断电保存全局变量.vi" "总磷自动测试量程配置"() -> (w482:T13)
        n248 = global read "总磷总氮断电保存全局变量.vi" "总磷消解时长"() -> (w481:dbl)
      }
      frame 2 {
        n249 = Unbundle By Name(w487) -> ("总氮跨度值"=w486:dbl, "总氮零点标准液浓度"=w485:dbl, "总氮跨度标准液浓度"=w484:dbl, "总氮标准液标准浓度"=w483:dbl)
        n250 = global read "总磷总氮断电保存全局变量.vi" "总氮自动测试量程配置"() -> (w489:T13)
        n251 = global read "总磷总氮断电保存全局变量.vi" "总氮消解时长"() -> (w488:dbl)
      }
      frame 3 {
        n252 = Unbundle By Name(w494) -> ("氨氮跨度值"=w493:dbl, "氨氮零点标准液浓度"=w492:dbl, "氨氮跨度标准液浓度"=w491:dbl, "氨氮标准液标准浓度"=w490:dbl)
        n253 = global read "总磷总氮断电保存全局变量.vi" "氨氮自动测试量程配置"() -> (w495:T13)
      }
      frame 4 {
        n254 = Unbundle By Name(w500) -> ("磷酸盐跨度值"=w499:dbl, "磷酸盐零点标准液浓度"=w498:dbl, "磷酸盐跨度标准液浓度"=w497:dbl, "磷酸盐标准液标准浓度"=w496:dbl)
        n255 = global read "总磷总氮断电保存全局变量.vi" "磷酸盐自动测试量程配置"() -> (w501:T13)
      }
      frame 5 {
        n256 = Unbundle By Name(w506) -> ("硝氮跨度值"=w505:dbl, "硝氮零点标准液浓度"=w504:dbl, "硝氮跨度标准液浓度"=w503:dbl, "硝氮标准液标准浓度"=w502:dbl)
        n257 = global read "总磷总氮断电保存全局变量.vi" "硝氮自动测试量程配置"() -> (w507:T13)
      }
      frame 6 {
        n258 = Unbundle By Name(w512) -> ("亚硝氮跨度值"=w511:dbl, "亚硝氮零点标准液浓度"=w510:dbl, "亚硝氮跨度标准液浓度"=w509:dbl, "亚硝氮标准液标准浓度"=w508:dbl)
        n259 = global read "总磷总氮断电保存全局变量.vi" "亚硝氮自动测试量程配置"() -> (w513:T13)
      }
      frame 7 {
        n260 = Unbundle By Name(w518) -> ("硅酸盐跨度值"=w517:dbl, "硅酸盐零点标准液浓度"=w516:dbl, "硅酸盐跨度标准液浓度"=w515:dbl, "硅酸盐标准液标准浓度"=w514:dbl)
        n261 = global read "总磷总氮断电保存全局变量.vi" "硅酸盐自动测试量程配置"() -> (w519:T13)
      }
      frame 8 {
        n262 = Unbundle By Name(w524) -> ("硫化物跨度值"=w523:dbl, "硫化物零点标准液浓度"=w522:dbl, "硫化物跨度标准液浓度"=w521:dbl, "硫化物标准液标准浓度"=w520:dbl)
        n263 = global read "总磷总氮断电保存全局变量.vi" "硫化物自动测试量程配置"() -> (w525:T13)
      }
      frame 22 {
        n264 = Unbundle By Name(w530) -> ("COD跨度值"=w529:dbl, "COD零点标准液浓度"=w528:dbl, "COD跨度标准液浓度"=w527:dbl, "COD标准液标准浓度"=w526:dbl)
        n265 = global read "总磷总氮断电保存全局变量.vi" "COD自动测试量程配置"() -> (w532:T13)
        n266 = global read "总磷总氮断电保存全局变量.vi" "CODcr消解时长"() -> (w531:dbl)
      }
    }
    "消解时长" <- w462
    n267 = local write "盐度自动补偿："(w469) -> ()
    n268 = local write "跨度值"(w464) -> ()
    n269 = local write "零点核查标液浓度"(w465) -> ()
    n270 = local write "跨度核查标液浓度"(w466) -> ()
    n271 = local write "标样核查标液浓度"(w467) -> ()
    n272 = To Unsigned Word Integer(number=w461) -> (unsigned 16bit integer=w460:T14)
    n273 = Unbundle By Name(w460) -> ("水样测试量程模式"=w459:u16, "空白核查量程模式"=w457:u16, "跨度核查量程模式"=w456:u16, "加标回收量程模式"=w455:u16, "标样核查量程模式"=w458:u16)
    n274 = local write "水样测试量程模式"(w459) -> ()
    n275 = local write "零点核查量程模式"(w457) -> ()
    n276 = local write "跨度核查量程模式"(w456) -> ()
    n277 = local write "加标回收量程模式"(w455) -> ()
    n278 = local write "标样核查量程模式"(w458) -> ()
  }
